vi "kf_init.vi"(0 "A":T1 format="%#_3g", 5 "B":T1 format="%#_3g", 7 "H":T1 format="%#_3g", 9 "x columns":i32=1) -> (4 "KF out":T2={"A"=[], "B"=[], "H"=[], "Q"=[], "R"=[], "x"=[], "P"=[], "x lim"=[], "y lim"=[], "K"=[], "Converge count"=-1} {"K" format="%#_3g"; "y lim" format="%#_3g"; "x lim" format="%#_3g"; "P" format="%#_3g"; "H" format="%#_3g"; "x" format="%#_3g"; "Q" format="%#_3g"; "R" format="%#_3g"; "B" format="%#_3g"; "A" format="%#_3g"})   [LabVIEW 2014]
uses:
  kalman_filter.ctl
  <vilib>/Analysis/Matrix/Datatypes/RealMatrix.ctl
  <vilib>/Analysis/Matrix/NI_Matrix.lvlib
panel:
  # "State transition matrix"
  # "Command response (from u).  Default is zeros."
  # "Map from measurement vector to state vector"
  # "Number of identical filters."
  # "Initialize a Kalman Filter from A, B and H matrices.   This sets all of the other elements to matrices of the correct size.   If B is empty, it is defaulted to zeros.  The covariances are initialized to zero because we don't know what value would be \"large\".   The measurement and process noises must be specified with kf_set_params, and when this is done, it will set the state covariance to the measurement noise if it is zero.   Similarly, x is initialized to zeros, with the specified number of columns.  If kf_set_parms is used with \"Initial measurement\", then the state created here is overwritten, and does not matter."
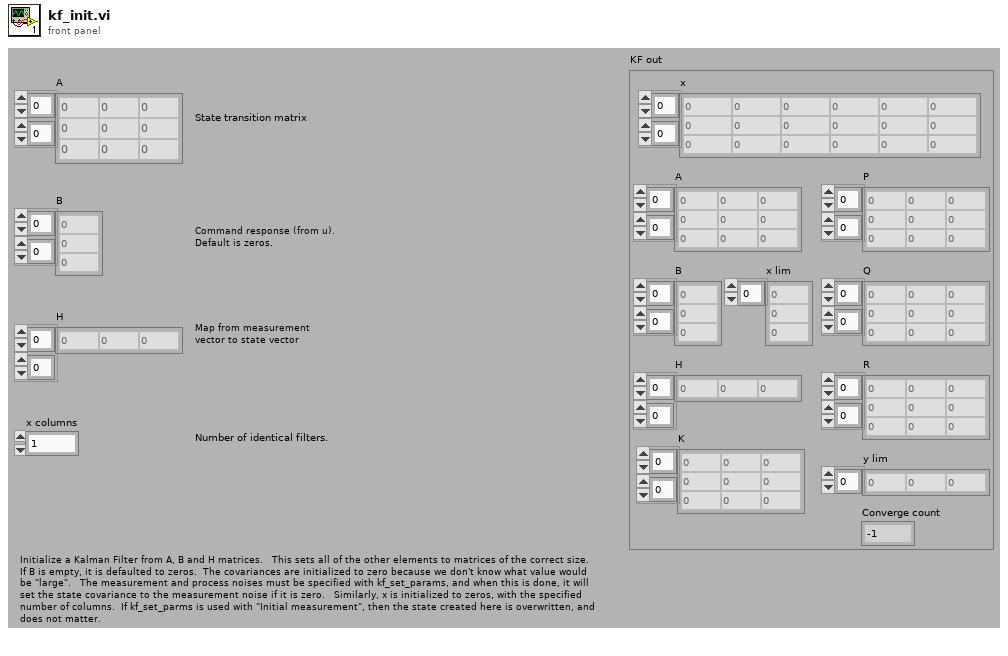
[diagram p1: front panel]
types:
  T1 = typedef "NI_Matrix.lvlib/RealMatrix.ctl" = dbl[][]
  T2 = typedef "kalman_filter.ctl" = cluster{"A":T1, "B":T1, "H":T1, "Q":T1, "R":T1, "x":T1, "P":T1, "x lim":dbl[], "y lim":dbl[], "K":T1, "Converge count":i32}
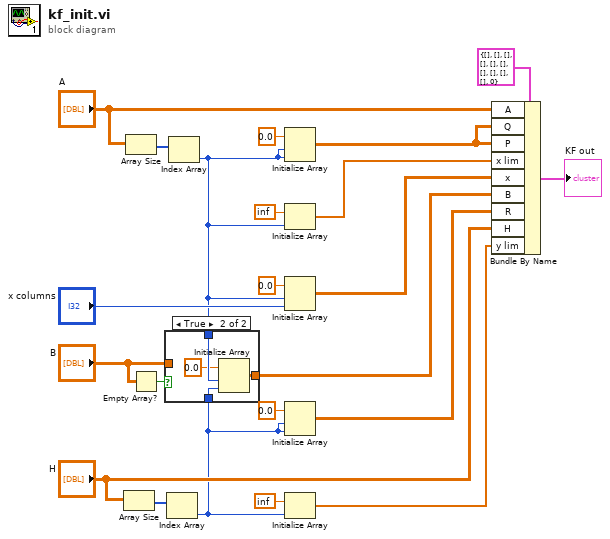
[diagram p0: block diagram]
diagram:
  n1 = Array Size(array="H") -> (size(s)=w16:i32[])
  n2 = Array Size(array="A") -> (size(s)=w20:i32[])
  n3 = Empty Array?(array="B") -> (empty?=w2:bool)
  n4 = Index Array(array=w16) -> (element=w4:i32)  [unwired: 1 in]
  n5 = Index Array(array=w20) -> (element=w5:i32)  [unwired: 1 in]
  n6 = case shown="True" w2 {
    tunnel: w5 -> [_ w27]
    tunnel: w4 -> [_ w26]
    tunnel: [w23 w24] -> w3
    tunnel: "B" -> [w23 _]
    frame False {
    }
    frame True {
      n7 = Initialize Array(0.0 ("element"), w27, w26) -> (w24:dbl[][])
    }
  }
  n8 = Initialize Array(0.0 ("Real Matrix Element"), w5, w5) -> (w9:dbl[][])
  n9 = Initialize Array(inf, w5) -> (w18:dbl[])
  n10 = Initialize Array(0.0 ("Real Matrix Element"), w5, "x columns") -> (w11:dbl[][])
  n11 = Initialize Array(0.0 ("Real Matrix Element"), w4, w4) -> (w6:dbl[][])
  n12 = Initialize Array(inf, w4) -> (w14:dbl[])
  n13 = Bundle By Name(cluster=T2 {"A"=[], "B"=[], "H"=[], "Q"=[], "R"=[], "x"=[], "P"=[], "x lim"=[], "y lim"=[], "K"=[], "Converge count"=0} ("KF in"), "A"="A", "Q"=w9, "P"=w9, "x lim"=w18, "x"=w11, "B"=w3, "R"=w6, "H"="H", "y lim"=w14) -> (→"KF out":T2)
